vi "TC560-Wait For Read.vi"(8 "error in":errorcluster) -> (0 "error out":errorcluster)   [LabVIEW 2018]
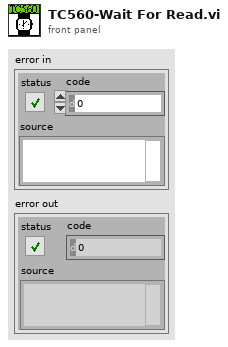
[diagram p1: front panel]
types:
  T1 = typedef "TC560-Configuration.ctl" = cluster{"Connection Setting":T2, "Wait For Read":u32}
  T2 = typedef "TC560-Connection Setting.ctl" = cluster{"VISA Resource Name":refnum<visa-resource-name>, "Baud Rate":u32, "Parity":u16, "Flow Control":u16}
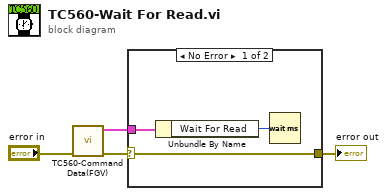
[diagram p0: block diagram]
diagram:
  n1 = call "TC560-Command Data(FGV).vi"("error in"="error in") -> ("error out"=w3:errorcluster, "Configuration Out"=w2:T1)  [unwired: 9 in]
  n2 = case shown="No Error" w3 {
    selector: w3 -> [w5 w8]
    tunnel: w2 -> [w7 _]
    tunnel: [w5 w8] -> w1
    frame No Error {
      n3 = Unbundle By Name(w7) -> ("Wait For Read"=w6:u32)
      n4 = Wait (ms)(milliseconds to wait=w6) -> ()  [unwired: 1 out]
    }
    frame Error {
    }
  }
  "error out" <- w1
